vi "insert_test.vi"(8 "error in (no error)":errorcluster, 10 "Test":T1, 11 "DB Session ID":i32) -> (0 "error out":errorcluster, 3 "DB Session ID out":i32)   [LabVIEW 2017, in "Database.lvlib"]
uses:
  Database.lvlib
  DB Test.ctl
  bin/Database.dll
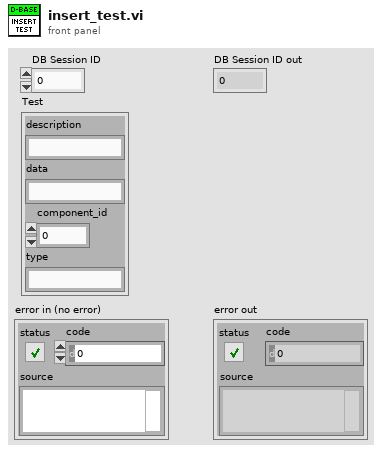
[diagram p1: front panel]
types:
  T1 = typedef "Database.lvlib/DB Test.ctl" = cluster{"description":string, "data":string, "component_id":i32, "type":string}
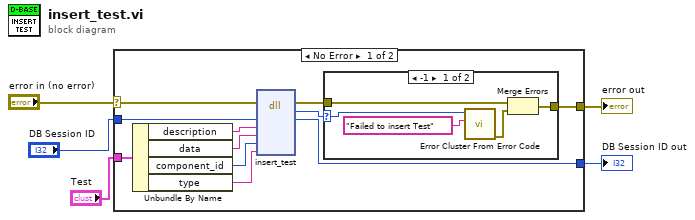
[diagram p0: block diagram]
diagram:
  n1 = case shown="No Error" "error in (no error)" {
    selector: "error in (no error)" -> [w14 w24]
    tunnel: [w13 w24] -> w3
    tunnel: "DB Session ID" -> [w15 w23]
    tunnel: [w12 w23] -> w2
    tunnel: "Test" -> [w11 _]
    frame No Error {
      n2 = Unbundle By Name(w11) -> ("description"=w10:string, "data"=w9:string, "component_id"=w8:i32, "type"=w7:string)
      n3 = dll-call lib="C:/Users/Caleb/Desktop/nebraska-silicon-lab/pixel-gantry-extra/LV/bin/Database.dll" fn="insert_test"(error in=w14, "conn_id"=w15, "description"=w10, "data"=w9, "component_id"=w8, "type"=w7) -> (error out=w16:errorcluster, "return type"=w6:i32, "conn_id"=w12:i32)  [unwired: 6 in, 1 out]
      n4 = case shown="-1" w6 {
        selector: w6 -> [w17 _]
        tunnel: w16 -> [w21 w22]
        tunnel: [w20 w22] -> w13
        frame -1 {
          n5 = call <vilib>:"Error Cluster From Error Code.vi"("error message (\"\")"="Failed to insert Test" ("error message (\"\")"), "error code (0)"=w17) -> ("error out"=w19:errorcluster)  [unwired: 7 in]
          n6 = Merge Errors(w21, w19) -> (w20:errorcluster)
        }
        frame Default {
          # "Ok"
        }
      }
    }
    frame Error {
    }
  }
  "error out" <- w3
  "DB Session ID out" <- w2
